vi "Get Item at Grid Point.vi"(8 "error in":errorcluster, 10 "Location":cluster{"X":i32, "Y":i32}, 11 "SourceGrid in":refnum<class "SourceGrid.lvclass">) -> (0 "error out":errorcluster, 1 "Cell Position":cluster{"Row":i32, "Column":i32}, 2 "Cell out":refnum<class "Cell.lvclass">, 3 "SourceGrid out":refnum<class "SourceGrid.lvclass">)   [LabVIEW 2024, in "SourceGrid.lvlib" / "SourceGrid.lvclass"]
uses:
  SourceGrid.lvclass
  Cells/Cell/Cell.lvclass
  SourceGrid.lvclass/SourceGrid.ctl
  D:/git/Sourcegrid-LabVIEW/dll/SourceGrid.dll
  dll/SourceGrid.dll
  System.Windows.Forms
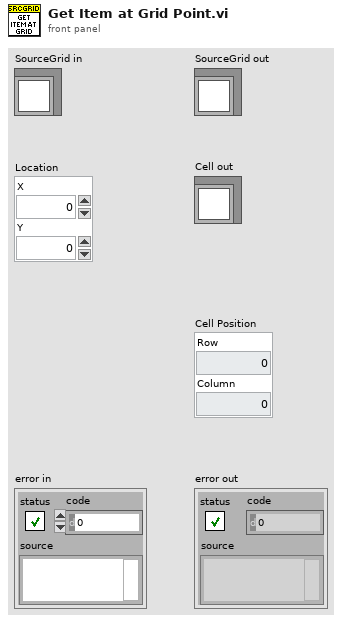
[diagram p1: front panel]
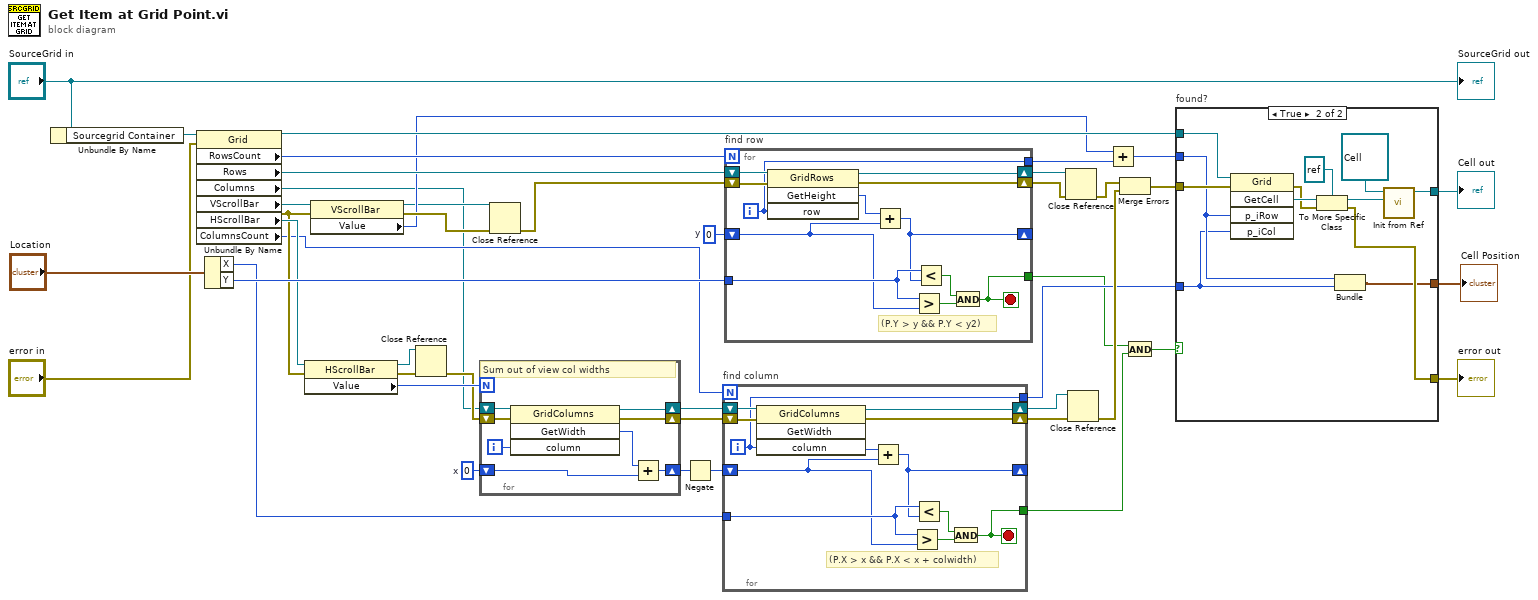
[diagram p0: block diagram]
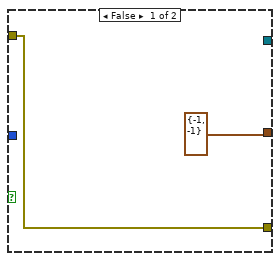
[diagram p2: hidden frame]
diagram:
  w33 = 0  # x
  w40 = 0  # y
  n1 = Unbundle By Name("SourceGrid in") -> ("Sourcegrid Container"=w43:refnum<k24>)
  n2 = property class="Grid"(reference=w43, error in="error in") -> (reference out=w29:refnum<k24>, error out=w20:errorcluster, "RowsCount"=w42:i32, "Rows"=w41:refnum<k24>, "Columns"=w8:refnum<k24>, "VScrollBar"=w21:refnum<k24>, "HScrollBar"=w24:refnum<k24>, "ColumnsCount"=w9:i32)
  n3 = Unbundle By Name("Location") -> ("X"=w30:i32, "Y"=w38:i32)
  n4 = property class="HScrollBar"(reference=w24, error in=w20) -> (reference out=w22:refnum<k24>, error out=w28:errorcluster, "Value"=w34:i32)
  n5 = property class="VScrollBar"(reference=w21, error in=w20) -> (reference out=w16:refnum<k24>, error out=w19:errorcluster, "Value"=w18:i32)
  n6 = Close Reference(reference=w22, error in (no error)=w28) -> (error out=w23:errorcluster)
  n7 = for {
    N: w34 -> [_]
    shift-right: [w48] -> w32
    shift-left: w33 -> [w49]
    shift-right: [w46] -> w27
    shift-left: w23 -> [w47]
    shift-right: [w45] -> w7
    shift-left: w8 -> [w52]
    i -> [w51]
    # "Sum out of view col widths"
    n8 = invoke class="GridColumns" method="GetWidth"(reference=w52, error in=w47, "column"=w51) -> (reference out=w45:refnum<k24>, error out=w46:errorcluster, "GetWidth"=w50:i32)  [unwired: 1 in, 1 out]
    n9 = Add(x=w50, y=w49) -> (x+y=w48:i32)
  }
  n10 = Close Reference(reference=w16, error in (no error)=w19) -> (error out=w17:errorcluster)
  n11 = Negate(x=w32) -> (-x=w31:i32)
  n12 = for "find column" {
    N: w9 -> [_]
    shift-right: [w57] -> _
    shift-left: w31 -> [w58]
    tunnel: w30 -> [w61]
    tunnel: [w56] -> w5
    shift-right: [w55] -> w25
    shift-left: w27 -> [w64]
    shift-right: [w54] -> w12
    shift-left: w7 -> [w63]
    tunnel: [w53] -> w2
    i -> [w56]
    stop <- w53 stop-if-true
    # "(P.X > x && P.X < x + colwidth)"
    n13 = invoke class="GridColumns" method="GetWidth"(reference=w63, error in=w64, "column"=w56) -> (reference out=w54:refnum<k24>, error out=w55:errorcluster, "GetWidth"=w62:i32)  [unwired: 1 in, 1 out]
    n14 = Add(x=w62, y=w58) -> (x+y=w57:i32)
    n15 = Greater?(x=w61, y=w58) -> (0:w59:bool)
    n16 = Less?(x=w61, y=w57) -> (x < y?=w60:bool)
    n17 = And(x=w60, y=w59) -> (x .and. y?=w53:bool)
  }
  n18 = for "find row" {
    N: w42 -> [_]
    shift-right: [w69] -> _
    shift-left: w40 -> [w70]
    tunnel: w38 -> [w73]
    tunnel: [w68] -> w37
    shift-right: [w67] -> w36
    shift-left: w17 -> [w76]
    shift-right: [w66] -> w14
    shift-left: w41 -> [w75]
    tunnel: [w65] -> w3
    i -> [w68]
    stop <- w65 stop-if-true
    # "(P.Y > y && P.Y < y2)"
    n19 = invoke class="GridRows" method="GetHeight"(reference=w75, error in=w76, "row"=w68) -> (reference out=w66:refnum<k24>, error out=w67:errorcluster, "GetHeight"=w74:i32)  [unwired: 1 in, 1 out]
    n20 = Add(x=w74, y=w70) -> (x+y=w69:i32)
    n21 = Greater?(x=w73, y=w70) -> (0:w71:bool)
    n22 = Less?(x=w73, y=w69) -> (x < y?=w72:bool)
    n23 = And(x=w72, y=w71) -> (x .and. y?=w65:bool)
  }
  n24 = Close Reference(reference=w14, error in (no error)=w36) -> (error out=w15:errorcluster)
  n25 = Close Reference(reference=w12, error in (no error)=w25) -> (error out=w13:errorcluster)
  n26 = Add(x=w18, y=w37) -> (x+y=w6:i32)
  n27 = Merge Errors(w15, w13) -> (w26:errorcluster)
  n28 = And(x=w3, y=w2) -> (x .and. y?=w1:bool)
  n29 = case "found?" shown="True" w1 {
    tunnel: w29 -> [_ w90]
    tunnel: w26 -> [w78 w86]
    tunnel: [_ w84] -> w11
    tunnel: [w78 w83] -> w10
    tunnel: w6 -> [_ w81]
    tunnel: w5 -> [_ w80]
    tunnel: [cluster{i32, i32} {-1, -1} w79] -> w4
    frame False {
    }
    frame True {
      n30 = invoke class="Grid" method="GetCell"(reference=w90, error in=w86, "p_iRow"=w81, "p_iCol"=w80) -> (error out=w87:errorcluster, "GetCell"=w89:refnum<k24>)  [unwired: 1 in, 3 out]
      n31 = To More Specific Class(target class=refnum<k24> refnum ("Cell Ref"), reference=w89, error in=w87) -> (specific class reference=w85:refnum<k24>, error out=w83:errorcluster)
      n32 = Bundle(w81, w80) -> (w79:cluster{i32, i32})  [unwired: 1 in]
      n33 = call-dynamic "Init from Ref.vi"("Cell Ref"=w85, "Cell in"=refnum<class "Cell.lvclass"> refnum) -> ("Cell out"=w84:refnum<class "Cell.lvclass">)  [unwired: 9 in]
    }
  }
  "error out" <- w10
  "Cell out" <- w11
  "Cell Position" <- w4
  "SourceGrid out" <- "SourceGrid in"
